vi "NavX Angle Test.vi"(7 "Target Angle":dbl, 8 "Error In":errorcluster, 11 "RobotDriveDevRefnum":T1={"DevStatus"={"status"=FALSE, "code"=0, "source"=""}, "Motors[]"=[], "Square Inputs"=FALSE, "Max Output"=1.0}) -> (0 "error out":errorcluster, 2 "Motor Values":dbl[](array[numeric]), 3 "RobotDriveDevRef":T1={"DevStatus"={"status"=FALSE, "code"=0, "source"=""}, "Motors[]"=[], "Square Inputs"=FALSE, "Max Output"=1.0})   [LabVIEW 2015]
uses:
  <vilib>/Rock Robotics/WPI/RobotDrive/WPI_RobotDriveDevRef.ctl
  <vilib>/Rock Robotics/WPI/MotorControl/WPI_MotorControlDeviceRef.ctl
  <vilib>/Rock Robotics/WPI/MotorControl/WPI_MotorControlType.ctl
  <vilib>/Rock Robotics/SystemInterfaces/DIO/FPGA_DIOPWMChannel.ctl
  <vilib>/Rock Robotics/WPI/PWM/WPI_PWMDeadband.ctl
  <vilib>/Rock Robotics/WPI/CAN/Jaguar/SubVIs/WPI_CANJaguar_ControlMode.ctl
  <vilib>/Rock Robotics/WPI/CAN/TalonSRX/WPI_CANTalonSRX_APIControlMode.ctl
  Robot Global Data.vi
  <vilib>/Rock Robotics/WPI/RobotDrive/WPI_RobotDriveArcadeDrive_Standard(NoSaturation).vi
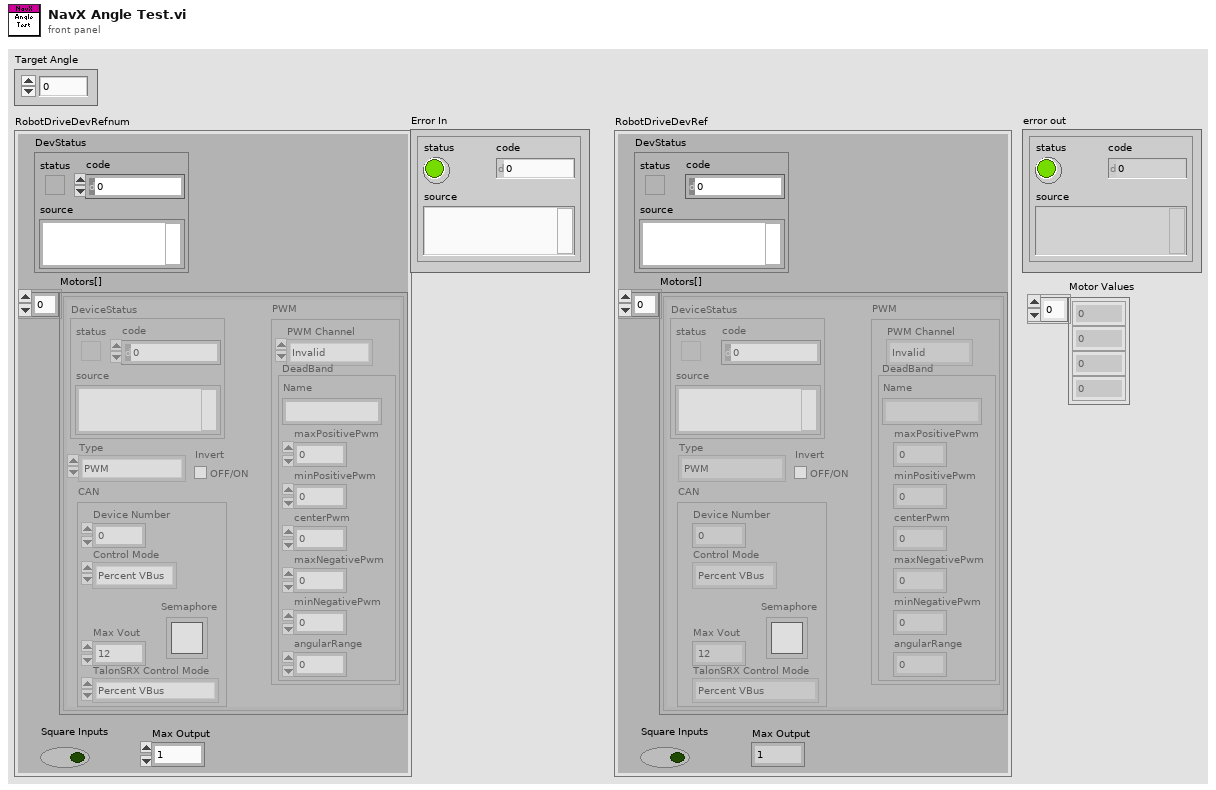
[diagram p1: front panel]
types:
  T1 = typedef "WPI_RobotDriveDevRef.ctl" = cluster{"DevStatus":errorcluster, "Motors[]":T2[], "Square Inputs":bool, "Max Output":dbl}
  T2 = typedef "WPI_MotorControlDeviceRef.ctl" = cluster{"DeviceStatus":errorcluster, "Type":T3, "PWM":cluster{"PWM Channel":T4, "DeadBand":T5}, "CAN":cluster{"Device Number":u8, "Control Mode":T6, "Semaphore":T7, "Max Vout":dbl, "TalonSRX Control Mode":T8}, "Invert":bool}
  T3 = typedef "WPI_MotorControlType.ctl" = enum16{"PWM", "CAN", "CANTalonSRX"}
  T4 = typedef "FPGA_DIOPWMChannel.ctl" = enum8{"PWM 0", "PWM 1", "PWM 2", "PWM 3", "PWM 4", "PWM 5", "PWM 6", "PWM 7", "PWM 8", "PWM 9", "PWM MXP 0", "PWM MXP 1", "PWM MXP 2", "PWM MXP 3", "PWM MXP 4", "PWM MXP 5", "PWM MXP 6", "PWM MXP 7", "PWM MXP 8", "PWM MXP 9", "Invalid"}
  T5 = typedef "WPI_PWMDeadband.ctl" = cluster{"Name":string, "maxPositivePwm":i32, "minPositivePwm":i32, "centerPwm":i32, "maxNegativePwm":i32, "minNegativePwm":i32, "angularRange":u16}
  T6 = typedef "WPI_CANJaguar_ControlMode.ctl" = enum8{"Percent VBus", "Current", "Speed", "Position", "Voltage"}
  T7 = typedef "Semaphore RefNum" = refnum<k1>
  T8 = typedef "WPI_CANTalonSRX_APIControlMode.ctl" = enum8{"Percent VBus", "Speed", "Position", "Slave", "Unchanged / Invalid", "Voltage Compensation", "Current", "Motion Profile"}
  T9 = cluster{"Yaw":dbl, "Roll":dbl, "Pitch":dbl, "Heading":dbl, "Fused Heading":dbl}
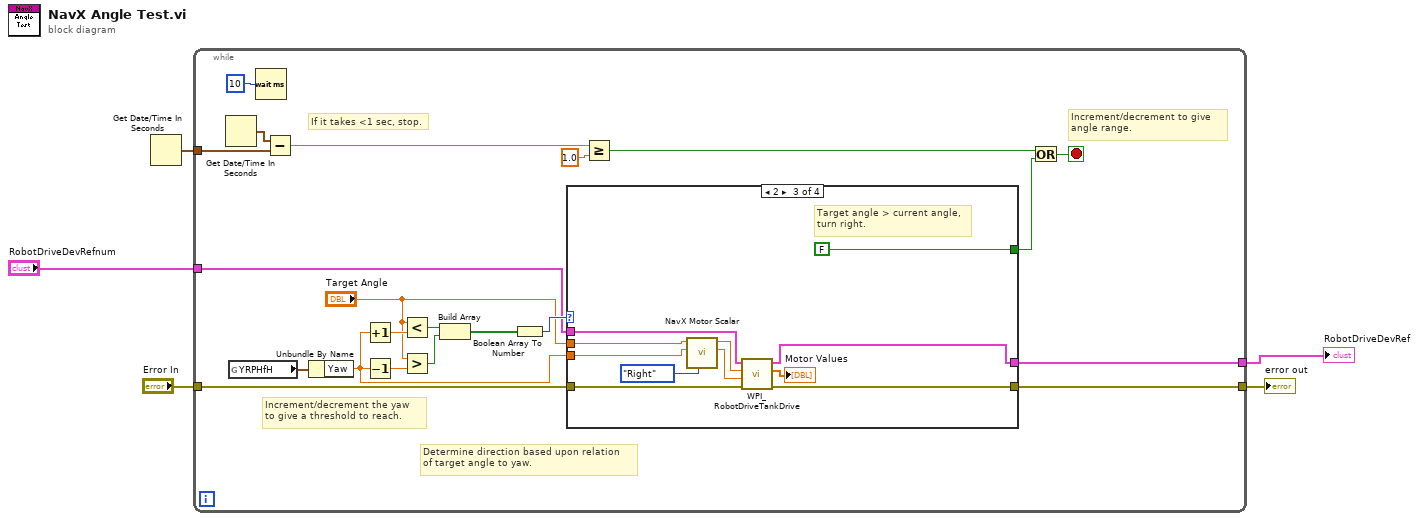
[diagram p0: block diagram]
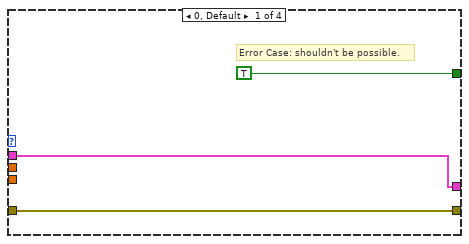
[diagram p2: hidden frame]
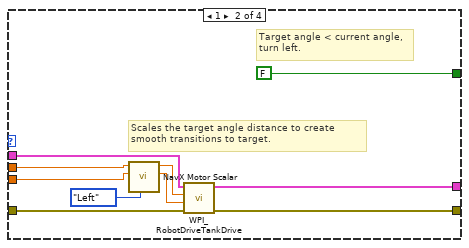
[diagram p3: hidden frame]
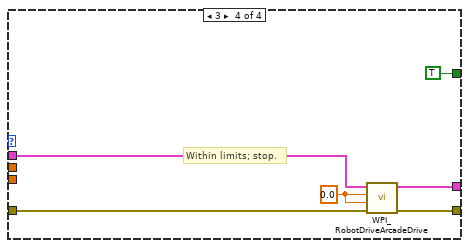
[diagram p4: hidden frame]
diagram:
  n1 = Get Date/Time In Seconds() -> (seconds since 1Jan1904=w1:timestamp)
  n2 = while {
    tunnel: "RobotDriveDevRefnum" -> [w19]
    tunnel: "Error In" -> [w18]
    tunnel: [w17] -> w5
    tunnel: [w16] -> w2
    tunnel: w1 -> [w10]
    stop <- w11 stop-if-true
    # "If it takes <1 sec, stop."
    # "Determine direction based upon relation\nof target angle to yaw."
    # "Increment/decrement the yaw\nto give a threshold to reach."
    # "Increment/decrement to give\nangle range."
    n3 = Get Date/Time In Seconds() -> (seconds since 1Jan1904=w9:timestamp)
    n4 = global read "Robot Global Data.vi" "YRPHfH"() -> (w14:T9)
    n5 = Wait (ms)(milliseconds to wait=u32 10) -> ()  [unwired: 1 out]
    n6 = Subtract(x=w9, y=w10) -> (x-y=w8:dbl)
    n7 = Unbundle By Name(w14) -> ("Yaw"=w12:dbl)
    n8 = Increment(x=w12) -> (x+1=w24:dbl)
    n9 = Decrement(x=w12) -> (x-1=w25:dbl)
    n10 = Less?(x="Target Angle", y=w24) -> (x < y?=w22:bool)
    n11 = Greater?(x="Target Angle", y=w25) -> (0:w23:bool)
    n12 = Build Array(w22, w23) -> (w21:bool[])
    n13 = Boolean Array To Number(Boolean array=w21) -> (number=w20:u32)
    n14 = case shown="2" w20 {
      tunnel: w19 -> [w29 w39 w49 w55]
      tunnel: w18 -> [w28 w38 w48 w54]
      tunnel: [w29 w37 w46 w53] -> w17
      tunnel: [w28 w36 w47 w52] -> w16
      tunnel: [TRUE FALSE FALSE TRUE] -> w15
      tunnel: "Target Angle" -> [_ w33 w45 _]
      tunnel: w12 -> [_ w32 w44 _]
      frame 0, Default {
        # "Error Case: shouldn't be possible."
      }
      frame 1 {
        # "Scales the target angle distance to create smooth transitions to target."
        # "Target angle < current angle,\nturn left."
        n15 = call "NavX Motor Scalar.vi"("Direction"=enum16{"Left", "Right"}."Left", "Yaw"=w32, "Target Angle"=w33) -> ("Right Motor Out"=w30:dbl, "Left Motor Out"=w31:dbl)  [unwired: 7 in]
        n16 = call <vilib>:"WPI_RobotDriveTankDrive.vi"("error in (no error)"=w38, "Right axis value"=w30, "Left axis value"=w31, "RobotDriveDevRef"=w39) -> ("error out"=w36:errorcluster, "RobotDriveDevRef"=w37:T1)  [unwired: 5 in, 1 out]
      }
      frame 2 {
        # "Target angle > current angle,\nturn right."
        n17 = call "NavX Motor Scalar.vi"("Direction"=enum16{"Left", "Right"}."Right", "Yaw"=w44, "Target Angle"=w45) -> ("Right Motor Out"=w41:dbl, "Left Motor Out"=w42:dbl)  [unwired: 7 in]
        n18 = call <vilib>:"WPI_RobotDriveTankDrive.vi"("error in (no error)"=w48, "Right axis value"=w41, "Left axis value"=w42, "RobotDriveDevRef"=w49) -> ("error out"=w47:errorcluster, "Motor Values"=→"Motor Values":dbl[], "RobotDriveDevRef"=w46:T1)  [unwired: 5 in]
      }
      frame 3 {
        w51 = 0.0 ("X axis value")
        # "Within limits; stop."
        n19 = call-poly <vilib>:"WPI_RobotDriveArcadeDrive.vi"("error in (no error)"=w54, "Y axis value"=w51, "X axis value"=w51, "RobotDriveDevRef"=w55) -> ("error out"=w52:errorcluster, "RobotDriveDevRef"=w53:T1)  [unwired: 5 in, 1 out]
      }
    }
    n20 = Greater Or Equal?(x=w8, y=1.0) -> (x >= y?=w6:bool)
    n21 = Or(x=w6, y=w15) -> (x .or. y?=w11:bool)
  }
  "RobotDriveDevRef" <- w5
  "error out" <- w2
